vi "Set Up Dialog - Conductivity.vi"() -> ()   [LabVIEW 2012]
panel:
  out "Calibration Instructions":string="1. Connect the sensor to your myDAQ as shown in the diagram above.\n\n2. Calibrate the CMN-100 using calibration solutions with known conductivity values. Your test samples must be between the high and low values of your calibration solutions. For example: If the expected measurement range is 500uS to 900uS perform a 2 point calibration with 400uS and 1000uS solutions.\n"
  # "iWorx - Conductivity - Set Up"
  # "Conductivity sensor (CMN-100)"
  # "iWorx"
  # "Sensor"
  # "CMN - 100"
  # "myDAQ"
  # "Computer"
  # "Adaptor"
  # "Connection Diagram"
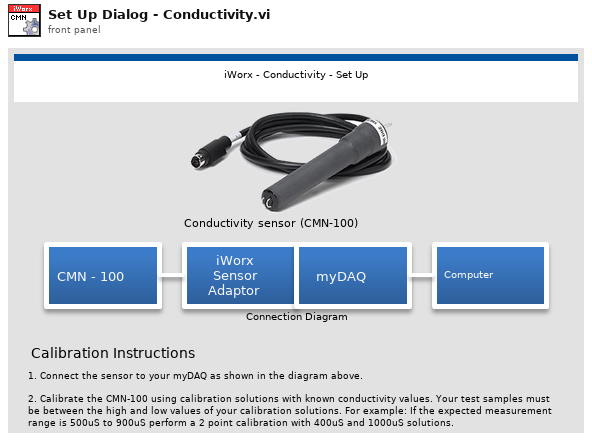
[diagram p1: front panel]
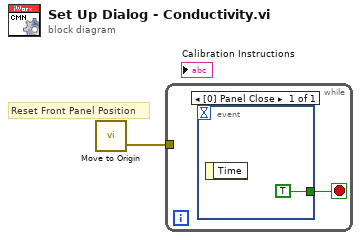
[diagram p0: block diagram]
diagram:
  # "Reset Front Panel Position"
  n1 = call "Move to Origin.vi"() -> ("Error Out"=w1:errorcluster)  [unwired: 3 in]
  n2 = while {
    tunnel: w1 -> [_]
    stop <- w2 stop-if-true
    n3 = event shown="[0] Panel Close" {
      selector: _ -> [_]
      dyn-events: _ -> [_]
      timeout: _ -> [_]
      tunnel: [TRUE] -> w2
      event Panel Close {
        n4 = event-data() -> ()  [unwired: 1 in, 1 out]
      }
    }
  }
